vi "PFI-28000-Chan-28144_Run Auto Balance.vi"(0 "PFI-28000-Chan-28144 in":refnum<class "PFI-28000-Chan-28144.lvclass">, 7 "Wait For Done":bool, 9 "Timeout":dbl format="%#_g sec", 11 "error in (no error)":errorcluster) -> (4 "PFI-28000-Chan-28144 out":refnum<class "PFI-28000-Chan-28144.lvclass">, 6 "Result":string, 15 "error out":errorcluster)   [LabVIEW 2017, in "PFI-28000-Chan-28144.lvclass"]
uses:
  PFI-28000-Chan-28144.lvclass
  C:/wc/07143 Precision Filters 28000 Support/Driver/source/Channel/PFI-28000-Channel.lvclass
  Utilities/PFI-28000-Utils.lvlib
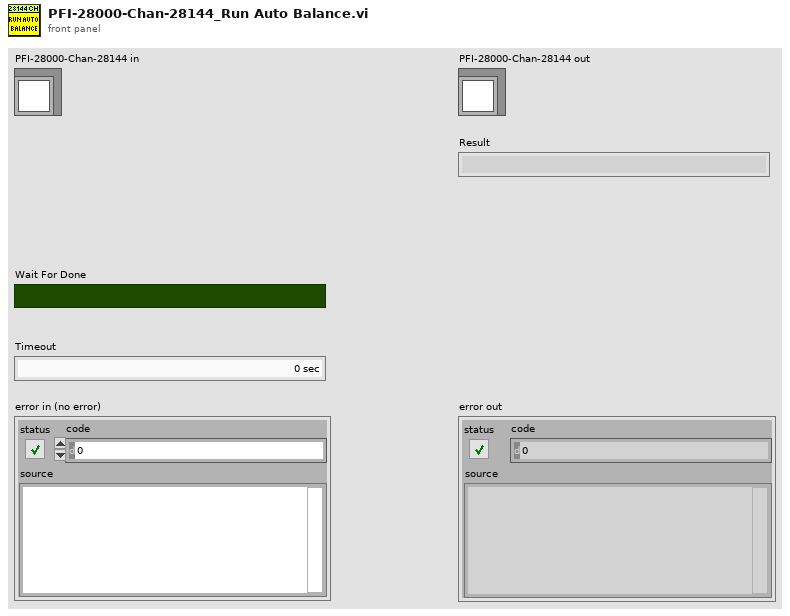
[diagram p1: front panel]
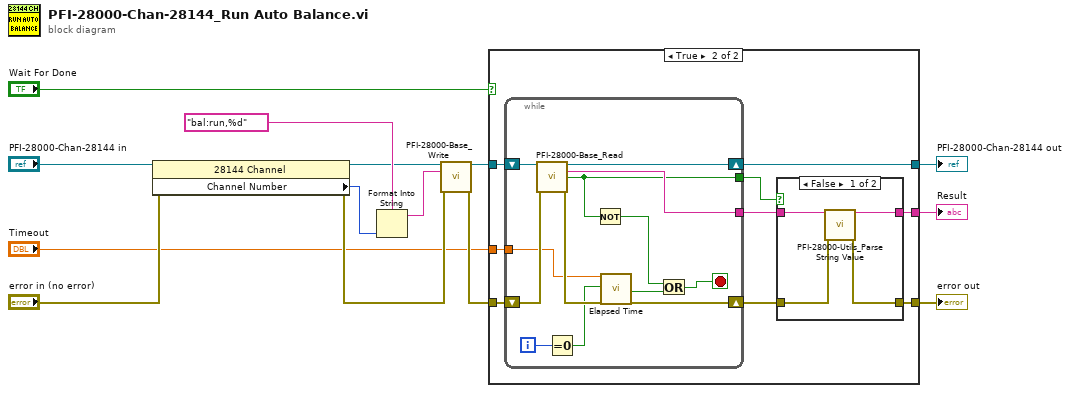
[diagram p0: block diagram]
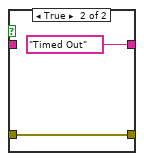
[diagram p3: hidden frame]
diagram:
  n1 = property class="28144 Channel"(reference="PFI-28000-Chan-28144 in", error in="error in (no error)") -> (reference out=w9:refnum<class "PFI-28000-Chan-28144.lvclass">, error out=w7:errorcluster, "Channel Number"=w13:i32)
  n2 = Format Into String(format string="bal:run,%d" ("empty string"), w13) -> (resulting string=w8:string)  [unwired: 2 in, 1 out]
  n3 = call-dynamic "PFI-28000-Base_Write.vi"("PFI-28000-Base in"=w9, "Command"=w8, "error in (no error)"=w7) -> ("PFI-28000-Base out"=w10:refnum<class "PFI-28000-Chan-28144.lvclass">, "error out"=w5:errorcluster)  [unwired: 11 in]
  n4 = case shown="True" "Wait For Done" {
    tunnel: w10 -> [w16 w25]
    tunnel: [w16 w24] -> w6
    tunnel: w5 -> [w15 w23]
    tunnel: "Timeout" -> [_ w22]
    tunnel: [w15 w19] -> w3
    tunnel: [_ w18] -> w2
    frame False {
    }
    frame True {
      n5 = while {
        shift-right: [w43] -> w24
        shift-left: w25 -> [w44]
        shift-right: [w40] -> w20
        shift-left: w23 -> [w42]
        tunnel: w22 -> [w39]
        tunnel: [w33] -> w21
        tunnel: [w32] -> w17
        i -> [w38]
        stop <- w35 stop-if-true
        n6 = call-dynamic "PFI-28000-Base_Read.vi"("PFI-28000-Base in"=w44, "error in (no error)"=w42) -> ("PFI-28000-Base out"=w43:refnum<class "PFI-28000-Chan-28144.lvclass">, "Response"=w33:string, "Timed Out"=w32:bool, "error out"=w41:errorcluster)  [unwired: 10 in]
        n7 = Equal To 0?(x=w38) -> (x = 0?=w37:bool)
        n8 = Not(x=w32) -> (.not. x?=w34:bool)
        n9 = call "Elapsed Time"("Time Target (s)"=w39, "Reset"=w37, "error in (no error)"=w41) -> ("Time has Elapsed"=w36:bool, "error out"=w40:errorcluster)  [unwired: 9 in, 6 out]
        n10 = Or(x=w34, y=w36) -> (x .or. y?=w35:bool)
      }
      n11 = case shown="False" w17 {
        tunnel: w21 -> [w29 _]
        tunnel: w20 -> [w28 w31]
        tunnel: [w27 w31] -> w19
        tunnel: [w26 "Timed Out" ("empty string")] -> w18
        frame False {
          n12 = call "PFI-28000-Utils_Parse String Value.vi"("String"=w29, "error in (no error)"=w28) -> ("String Value"=w26:string, "error out"=w27:errorcluster)  [unwired: 11 in, 1 out]
        }
        frame True {
        }
      }
    }
  }
  "error out" <- w3
  "PFI-28000-Chan-28144 out" <- w6
  "Result" <- w2
